vi "set_pattern_type.vi"(8 "error in (no error)":errorcluster, 10 "subpattern?":bool, 11 "FPGAWrapperMH120124RAPS_PXI7813R in":refnum<class "FPGAWrapperMH120124RAPS_PXI7813R.lvclass">) -> (0 "error out":errorcluster, 3 "FPGAWrapperMH120124RAPS_PXI7813R out":refnum<class "FPGAWrapperMH120124RAPS_PXI7813R.lvclass">)   [LabVIEW 2010, in "FPGAWrapperMH120124RAPS_PXI7813R.lvclass"]
uses:
  FPGAWrapperMH120124RAPS_PXI7813R.lvclass
  FPGAWrapperMH120124RAPS_PXI7813R.lvclass/FPGAWrapperMH120124RAPS_PXI7813R.ctl
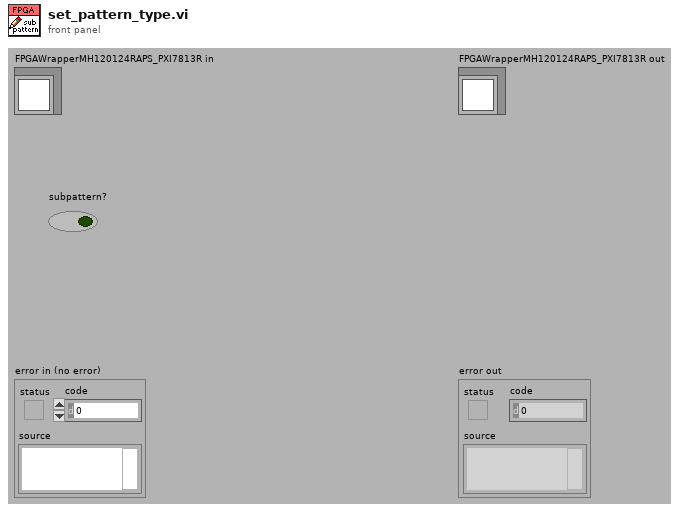
[diagram p1: front panel]
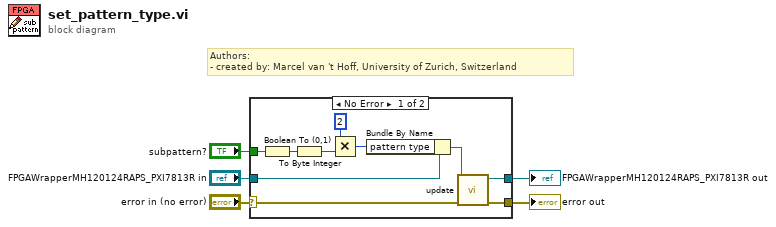
[diagram p0: block diagram]
diagram:
  # "Authors: \n- created by: Marcel van 't Hoff, University of Zurich, Switzerland"
  n1 = case shown="No Error" "error in (no error)" {
    selector: "error in (no error)" -> [w7 w17]
    tunnel: [w6 w17] -> w4
    tunnel: [w8 w16] -> w2
    tunnel: "FPGAWrapperMH120124RAPS_PXI7813R in" -> [w15 w16]
    tunnel: "subpattern?" -> [w14 _]
    frame No Error {
      n2 = Boolean To (0,1)(Boolean=w14) -> (0, 1=w13:i16)
      n3 = To Byte Integer(number=w13) -> (8bit integer=w10:i8)
      n4 = Multiply(x=i8 2 ("y"), y=w10) -> (x*y=w11:i8)
      n5 = Bundle By Name(cluster=w15, "pattern type"=w11) -> (w9:refnum<class "FPGAWrapperMH120124RAPS_PXI7813R.lvclass">)
      n6 = call-dynamic "update.vi"("error in (no error)"=w7, "FPGAWrapperMH120124RAPS_PXI7813R in"=w9) -> ("error out"=w6:errorcluster, "FPGAWrapperMH120124RAPS_PXI7813R out"=w8:refnum<class "FPGAWrapperMH120124RAPS_PXI7813R.lvclass">)  [unwired: 8 in]
    }
    frame Error {
    }
  }
  "error out" <- w4
  "FPGAWrapperMH120124RAPS_PXI7813R out" <- w2
